vi "GlobalNoteHandling.vi"() -> ()   [LabVIEW 2023]
panel:
  out "OUT_Gate_Closed":bool
  out "OUT_Intake_Beambreak":bool
  out "OUT_Shooter_Beambreak":bool
  out "OUT_ Intaking":bool
  out "OUT_Indexer":dbl
  out "REF_Indexer":string
  out "REF_Intake_2":string
  out "OUT_Intake_2":dbl
  out "OUT_Intake":dbl
  out "REF_Intake":string
  # "DEVICE REFERENCE NAMES"
  # "Outputs"
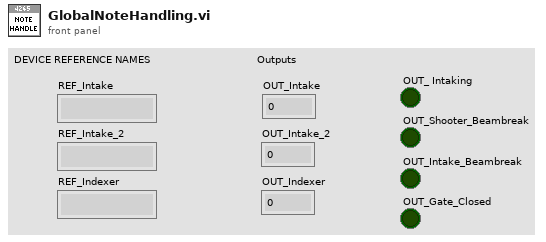
[diagram p1: front panel]
diagram:
